vi "ASM.StateFlow.vi"(8 "error in (no error)":errorcluster, 10 "StateToExecute":T1, 11 "ActorStateMachine in":refnum<class "ActorStateMachine.lvclass">) -> (0 "error out":errorcluster, 3 "ActorStateMachine out":refnum<class "ActorStateMachine.lvclass">)   [LabVIEW 2021, in "ActorStateMachine.lvlib" / "ActorStateMachine.lvclass"]
uses:
  ActorStateMachine.lvclass
  _ASM.State.ctl
  ActorStateMachine.lvclass/ActorStateMachine.ctl
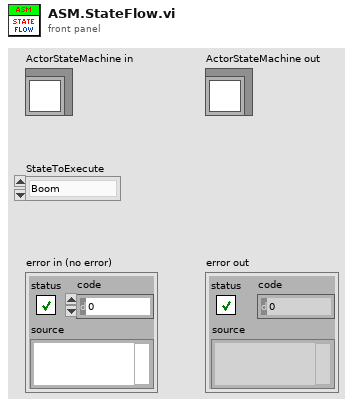
[diagram p1: front panel]
types:
  T1 = typedef "ActorStateMachine.lvlib/ActorStateMachine.lvclass/_ASM.State.ctl" = enum16{"Boom", "Pre-Init", "Init", "Post-Init", "Pre-Reset", "Reset", "Post-Reset", "Pre-Config", "Config", "Post-Config", "Pre-Ready", "Ready", "Post-Ready", "Pre-Running", "Running", "Next", "Post-Running", "Break", "Fail", "Crash", "Shutdown", "Doom"}
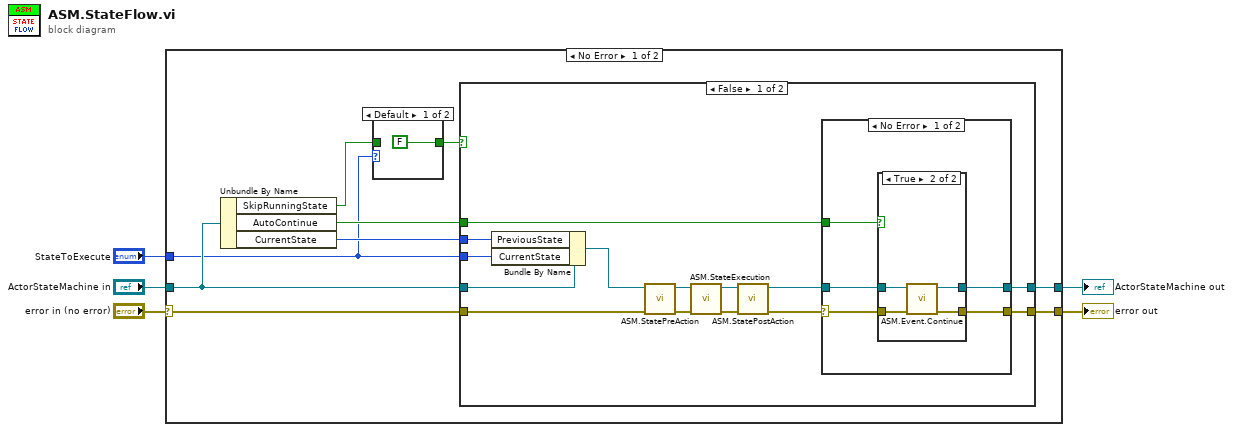
[diagram p0: block diagram]
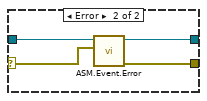
[diagram p4: hidden frame]
diagram:
  n1 = case shown="No Error" "error in (no error)" {
    selector: "error in (no error)" -> [w12 w49]
    tunnel: [w14 w49] -> w4
    tunnel: [w13 w48] -> w2
    tunnel: "ActorStateMachine in" -> [w11 w48]
    tunnel: "StateToExecute" -> [w8 _]
    frame No Error {
      n2 = Unbundle By Name(w11) -> ("SkipRunningState"=w7:bool, "AutoContinue"=w10:bool, "CurrentState"=w9:T1)
      n3 = case shown="Default" w8 {
        tunnel: w7 -> [_ w16]
        tunnel: [FALSE ("Break") w16] -> w6
        frame Default {
        }
        frame "Running" {
        }
      }
      n4 = case shown="False" w6 {
        tunnel: [w30 w46] -> w14
        tunnel: [w29 w47] -> w13
        tunnel: w12 -> [w28 w46]
        tunnel: w11 -> [w27 w47]
        tunnel: w10 -> [w26 _]
        tunnel: w8 -> [w25 _]
        tunnel: w9 -> [w24 _]
        frame False {
          n5 = Bundle By Name(cluster=w27, "PreviousState"=w24, "CurrentState"=w25) -> (w17:refnum<class "ActorStateMachine.lvclass">)
          n6 = call-dynamic "ASM.StatePreAction.vi"("error in (no error)"=w28, "ActorStateMachine in"=w17) -> ("error out"=w21:errorcluster, "ActorStateMachine out"=w23:refnum<class "ActorStateMachine.lvclass">)  [unwired: 8 in]
          n7 = call "ASM.StateExecution.vi"("error in (no error)"=w21, "ActorStateMachine in"=w23) -> ("error out"=w22:errorcluster, "ActorStateMachine out"=w19:refnum<class "ActorStateMachine.lvclass">)  [unwired: 8 in]
          n8 = call-dynamic "ASM.StatePostAction.vi"("error in (no error)"=w22, "ActorStateMachine in"=w19) -> ("error out"=w20:errorcluster, "ActorStateMachine out"=w18:refnum<class "ActorStateMachine.lvclass">)  [unwired: 8 in]
          n9 = case shown="No Error" w20 {
            selector: w20 -> [w35 w44]
            tunnel: [w32 w45] -> w30
            tunnel: w18 -> [w34 w43]
            tunnel: [w33 w42] -> w29
            tunnel: w26 -> [w31 _]
            frame No Error {
              n10 = case shown="True" w31 {
                tunnel: w35 -> [w37 w41]
                tunnel: [w37 w40] -> w32
                tunnel: w34 -> [w36 w39]
                tunnel: [w36 w38] -> w33
                frame False {
                }
                frame True {
                  n11 = call "ASM.Event.Continue.vi"("error in (no error)"=w41, "ActorStateMachine in"=w39) -> ("error out"=w40:errorcluster, "ActorStateMachine out"=w38:refnum<class "ActorStateMachine.lvclass">)  [unwired: 8 in]
                }
              }
            }
            frame Error {
              n12 = call "ASM.Event.Error.vi"("StateError"=w44, "ActorStateMachine in"=w43) -> ("error out"=w45:errorcluster, "ActorStateMachine out"=w42:refnum<class "ActorStateMachine.lvclass">)  [unwired: 8 in]
            }
          }
        }
        frame True {
        }
      }
    }
    frame Error {
    }
  }
  "error out" <- w4
  "ActorStateMachine out" <- w2
